vi "运维调试_CODCr.vi"() -> ()   [LabVIEW 2016, in "CodCr.lvlib"]
uses:
  CodCr.lvlib
  <vilib>/Utility/miscctls.llb/LVPointTypeDef.ctl
  <vilib>/Plasmionique/MB Master/MB_Master_Serial/MB_Master_Serial.lvclass
  C:/Program Files (x86)/National Instruments/LabVIEW 2016/vi.lib/Plasmionique/MB Master/MB_Master/MB_Master.lvclass
  <vilib>/Plasmionique/MB Master/MB Master.lvlib
  <vilib>/ptbypt/NI_PtbyPt.lvlib
panel:
  out "启动时间":timestamp format="%<%Y/%m/%d %H:%M:%S>T"
  out "?":errorcluster
  out "主循环次数":i32
  out "status":bool
  out "启动测量模式":T1(ring)
  out "曲线斜率B":sgl
  out "曲线斜率K":sgl
  out "量程上限":sgl
  out "量程下限":sgl
  out "消解时长":u16
  out "消解温度":u16
  out "测量精度":u16
  out "测量结果":sgl
  out "标样参考值":sgl
  out "量程":u16
  out "工作状态":T1(ring)
  out "仪器时间":timestamp format="%<%X\n%x>T"
  out "关键参数区":T2
  out "状态告警区":T3
  out "测量数据区":T4 {"单位" items=["ug/L", "mg/L", "ppm", "mg/m3", "cm", "ppb", "ug/m3", "%", "nmol/mol", "umol/mol", "MPN/L", "MPN/100ml", "ng/m3", "NTU", "无量纲", "ms/cm", "us/cm", "℃", "mV", "万个/L"]}
  out "error out":errorcluster
  out "系统时间":timestamp format="%<%Y/%m/%d %H:%M:%S>T"
  in  "VISA Resource":refnum<visa-resource-name>="COM9"
  out "Registers":u16[](array[numeric])
  in  "枚举":enum16{"读取", "写入", "读取参数"}(ring)
  in  "停止":bool
  in  "校时":bool
  in  "标样校准":bool
  in  "空白校准":bool
  in  "零点核查":bool
  in  "标样核查":bool
  in  "水样测试":bool
  in  "返回":bool
  in  "设置":bool
  # "mg/L"
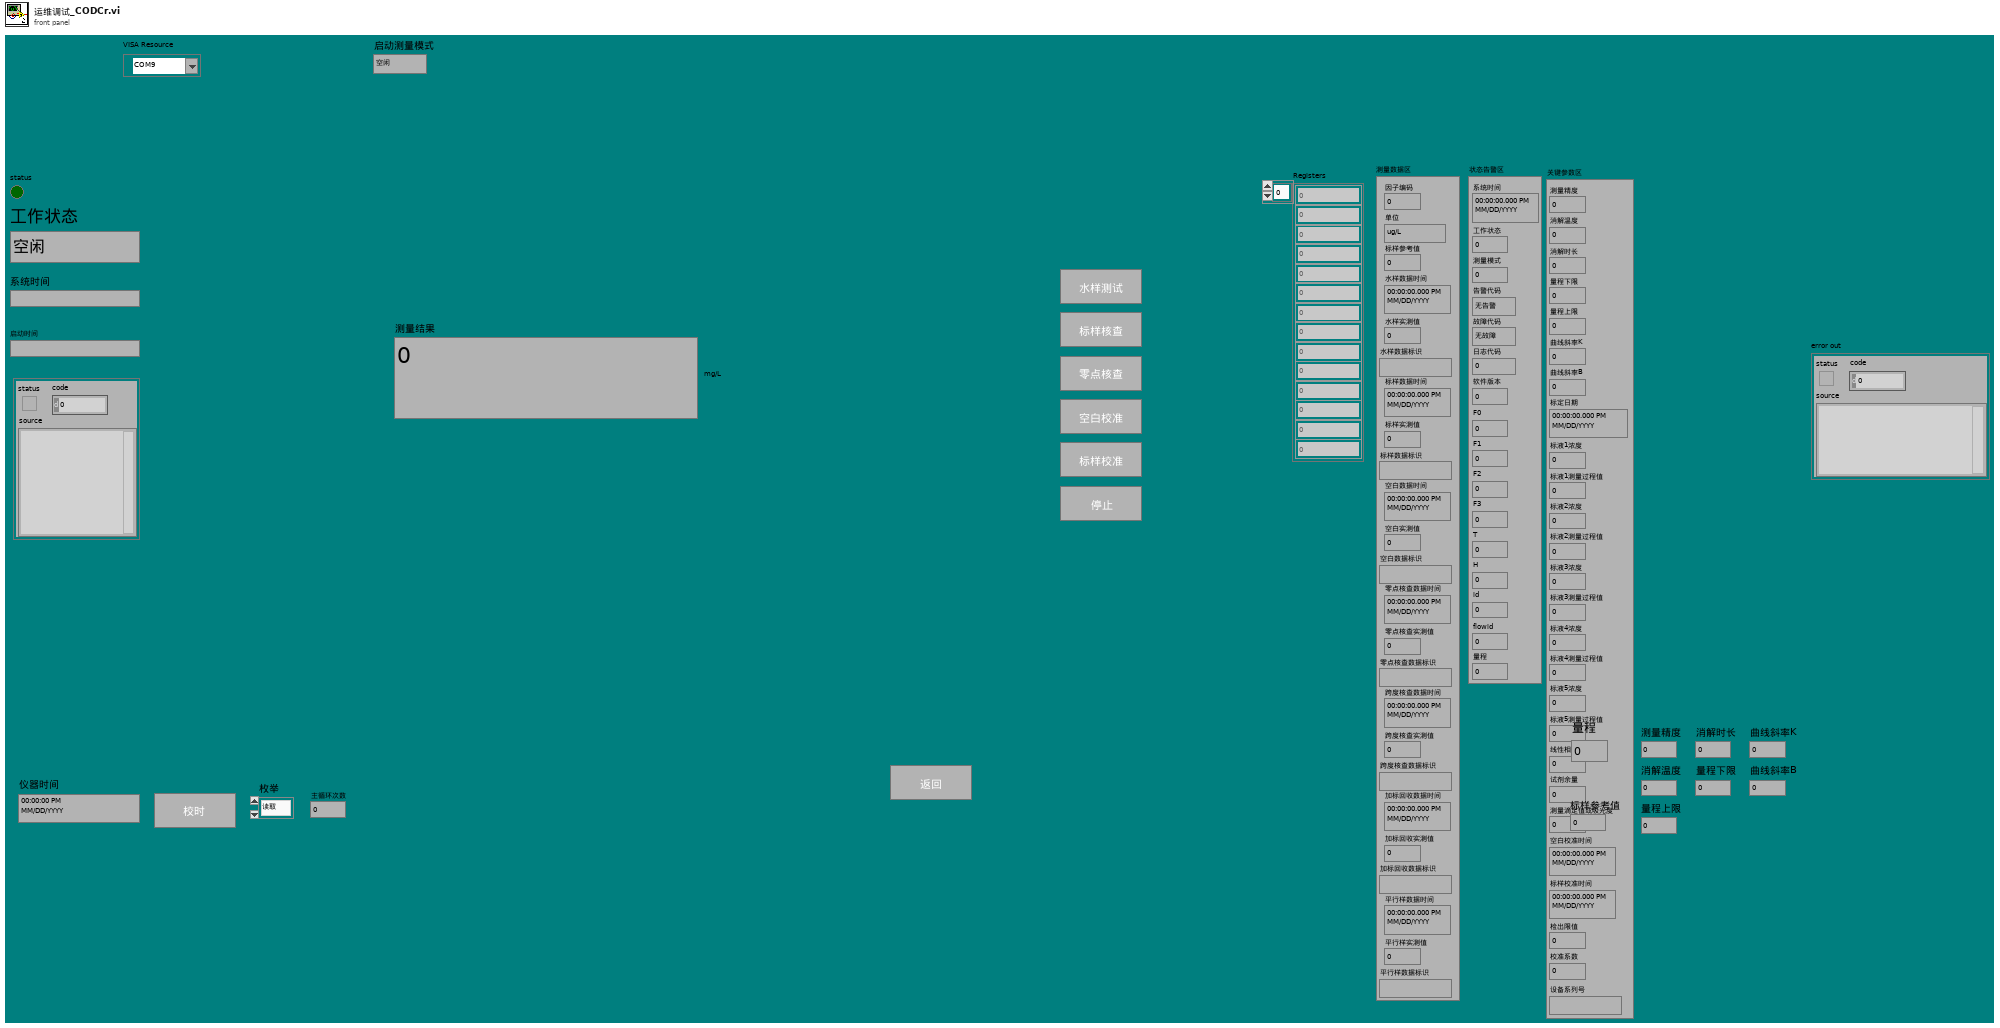
[diagram p1: front panel]
types:
  T1 = enum16{"空闲", "水样测试", "标样核查", "零点核查", "跨度核查", "空白测试", "平行样测试", "加标回收", "空白校准", "标样校准", "初始化（清洗）"}
  T2 = cluster{"测量精度":u16, "消解温度":u16, "消解时长":u16, "量程下限":sgl, "量程上限":sgl, "曲线斜率K":sgl, "曲线斜率B":sgl, "标定日期":timestamp, "标液1浓度":sgl, "标液1测量过程值":sgl, "标液2浓度":sgl, "标液2测量过程值":sgl, "标液3浓度":sgl, "标液3测量过程值":sgl, "标液4浓度":sgl, "标液4测量过程值":sgl, "标液5浓度":sgl, "标液5测量过程值":sgl, "线性相关系数":sgl, "试剂余量":u32, "测量滴定值或吸光度":sgl, "空白校准时间":timestamp, "标样校准时间":timestamp, "检出限值":sgl, "校准系数":sgl, "设备系列号":string}
  T3 = cluster{"系统时间":timestamp, "工作状态":u16, "测量模式":u16, "告警代码":enum16{"无告警", "缺试剂告警", "缺水样告警", "缺蒸馏水告警", "缺标液告警", "仪表漏液告警", "标定异常告警", "超量程告警", "加热异常", "低试剂预警", "超上限告警", "超下限告警", "仪表内部其他异常", "滴定异常告警", "电极异常告警", "量程切换告警", "参数设置告警", "PH电极电位异常", "电导率电极异常", "浊度光度异常", "溶解氧电极异常", "溶解氧光强异常", "温度异常告警", "PH异常告警", "溶解氧异常告警", "电导率异常告警", "浊度异常告警", "叶绿素异常告警", "藻密度异常告警", "蓝绿藻异常告警", "ORP异常告警", "氨氮异常告警", "清洁刷异常告警", "SD卡异常告警", "蓝牙异常告警", "Wifi异常告警", "流程异常告警"}, "故障代码":enum16{"无故障", "电机故障", "温度故障", "通讯故障", "滴定故障"}, "日志代码":u16, "软件版本":u16, "F0":sgl, "F1":sgl, "F2":sgl, "F3":sgl, "T":sgl, "H":sgl, "id":u16, "flowid":u16, "量程":u16}
  T4 = cluster{"因子编码":u32, "单位":u16, "标样参考值":sgl, "水样数据时间":timestamp, "水样实测值":sgl, "水样数据标识":string, "标样数据时间":timestamp, "标样实测值":sgl, "标样数据标识":string, "空白数据时间":timestamp, "空白实测值":sgl, "空白数据标识":string, "零点核查数据时间":timestamp, "零点核查实测值":sgl, "零点核查数据标识":string, "跨度核查数据时间":timestamp, "跨度核查实测值":sgl, "跨度核查数据标识":string, "加标回收数据时间":timestamp, "加标回收实测值":sgl, "加标回收数据标识":string, "平行样数据时间":timestamp, "平行样实测值":sgl, "平行样数据标识":string}
  T5 = cluster{"baud rate (bps)":u32, "stop bits":u16, "parity":u16, "flow control":u16, "timeout":u32, "retries":i32}
  T6 = cluster{"starting address":u16, "number of holding registers":u16}
  T7 = typedef "LVPointTypeDef.ctl" = cluster{"Horizontal":i16, "Vertical":i16}
  T8 = cluster{"时间标识":timestamp, "监测值":sgl, "单位":u16, "数据标识":string, "因子编码":u32, "标样参考值":sgl, "F0":sgl, "F1":sgl, "F2":sgl, "F3":sgl, "温度":sgl, "湿度":sgl, "量程标识":string}
  T9 = cluster{"系统时间":timestamp, "工作状态":enum16{"空闲", "水样测试", "标样核查", "零点核查", "跨度核查", "空白测试", "平行样测试", "加标回收", "空白校准", "标样校准", "初始化（清洗）"}, "测量模式":enum16{"待机", "连续模式", "周期模式", "定点模式", "受控模式", "手动模式"}, "告警代码":enum16{"无告警", "缺试剂告警", "缺水样告警", "缺蒸馏水告警", "缺标液告警", "仪表漏液告警", "标定异常告警", "超量程告警", "加热异常", "低试剂预警", "超上限告警", "超下限告警", "仪表内部其他异常", "滴定异常告警", "电极异常告警", "量程切换告警", "参数设置告警", "PH电极电位异常", "电导率电极异常", "浊度光度异常", "溶解氧电极异常", "溶解氧光强异常", "温度异常告警", "PH异常告警", "溶解氧异常告警", "电导率异常告警", "浊度异常告警", "叶绿素异常告警", "藻密度异常告警", "蓝绿藻异常告警", "ORP异常告警", "氨氮异常告警", "清洁刷异常告警", "SD卡异常告警", "蓝牙异常告警", "Wifi异常告警", "流程异常告警"}, "故障代码":enum16{"无故障", "电机故障", "温度故障", "通讯故障", "滴定故障"}, "日志代码":u16, "软件版本":u16, "F0":sgl, "F1":sgl, "F2":sgl, "F3":sgl, "T":sgl, "H":sgl, "id":u16, "flowid":u16, "量程":u16}
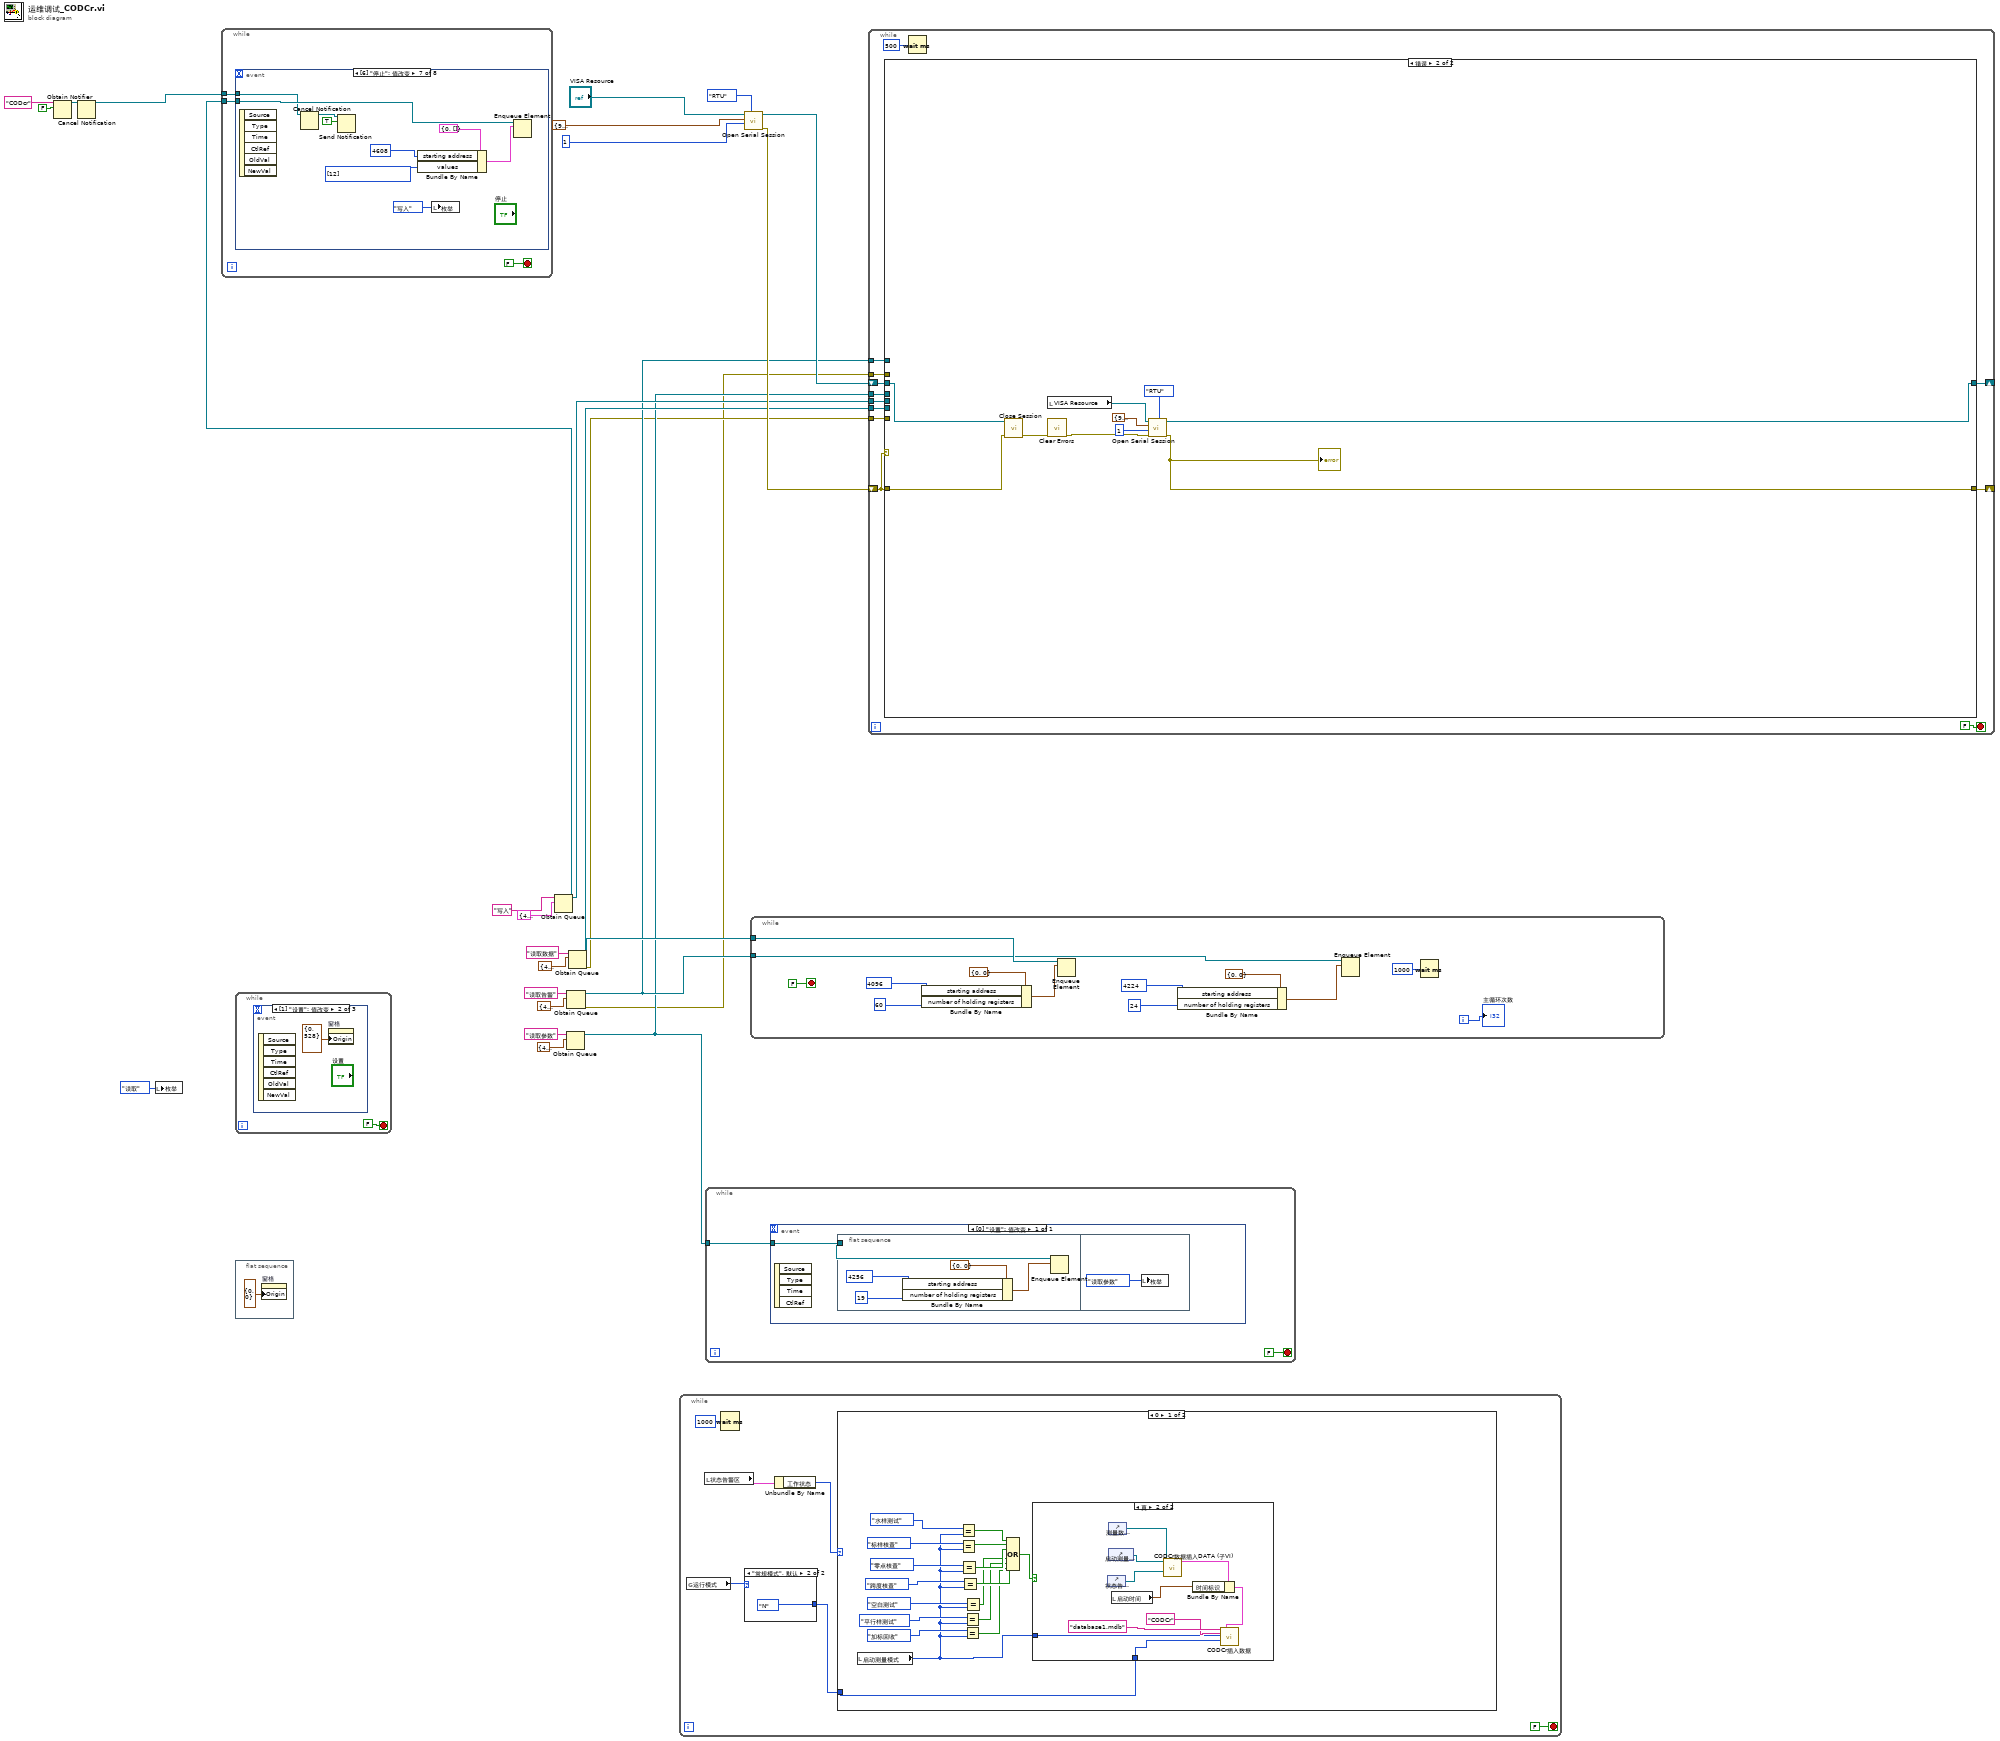
[diagram p0: block diagram]
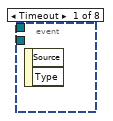
[diagram p2: hidden frame]
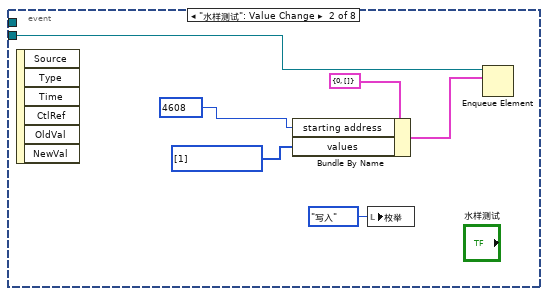
[diagram p3: hidden frame]
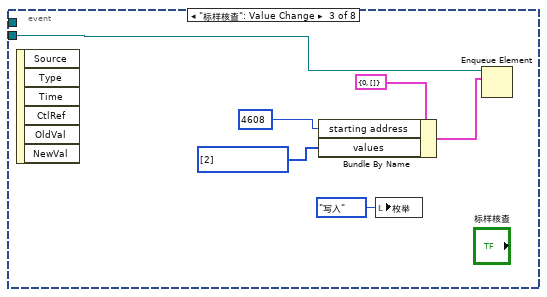
[diagram p4: hidden frame]
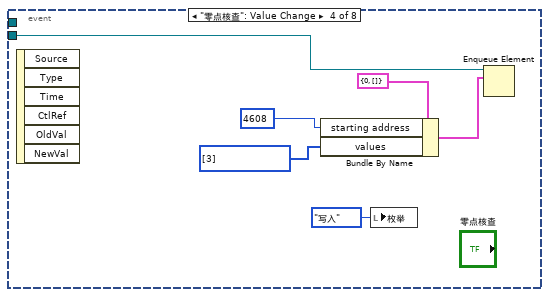
[diagram p5: hidden frame]
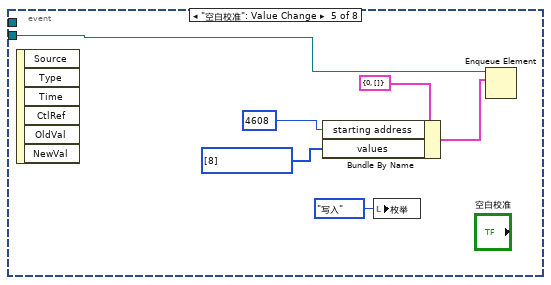
[diagram p6: hidden frame]
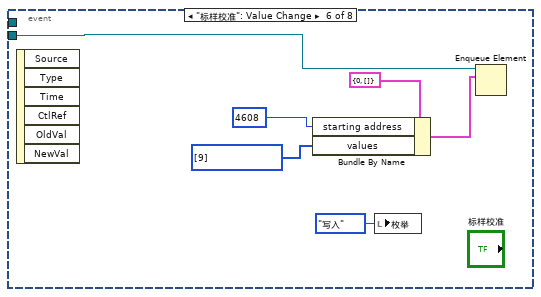
[diagram p7: hidden frame]
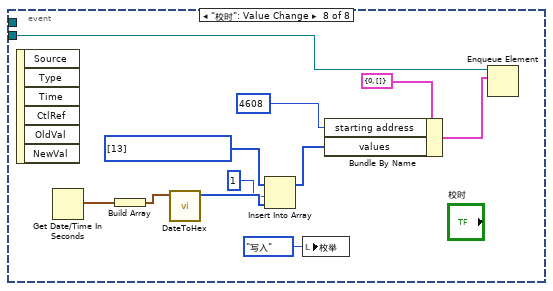
[diagram p8: hidden frame]
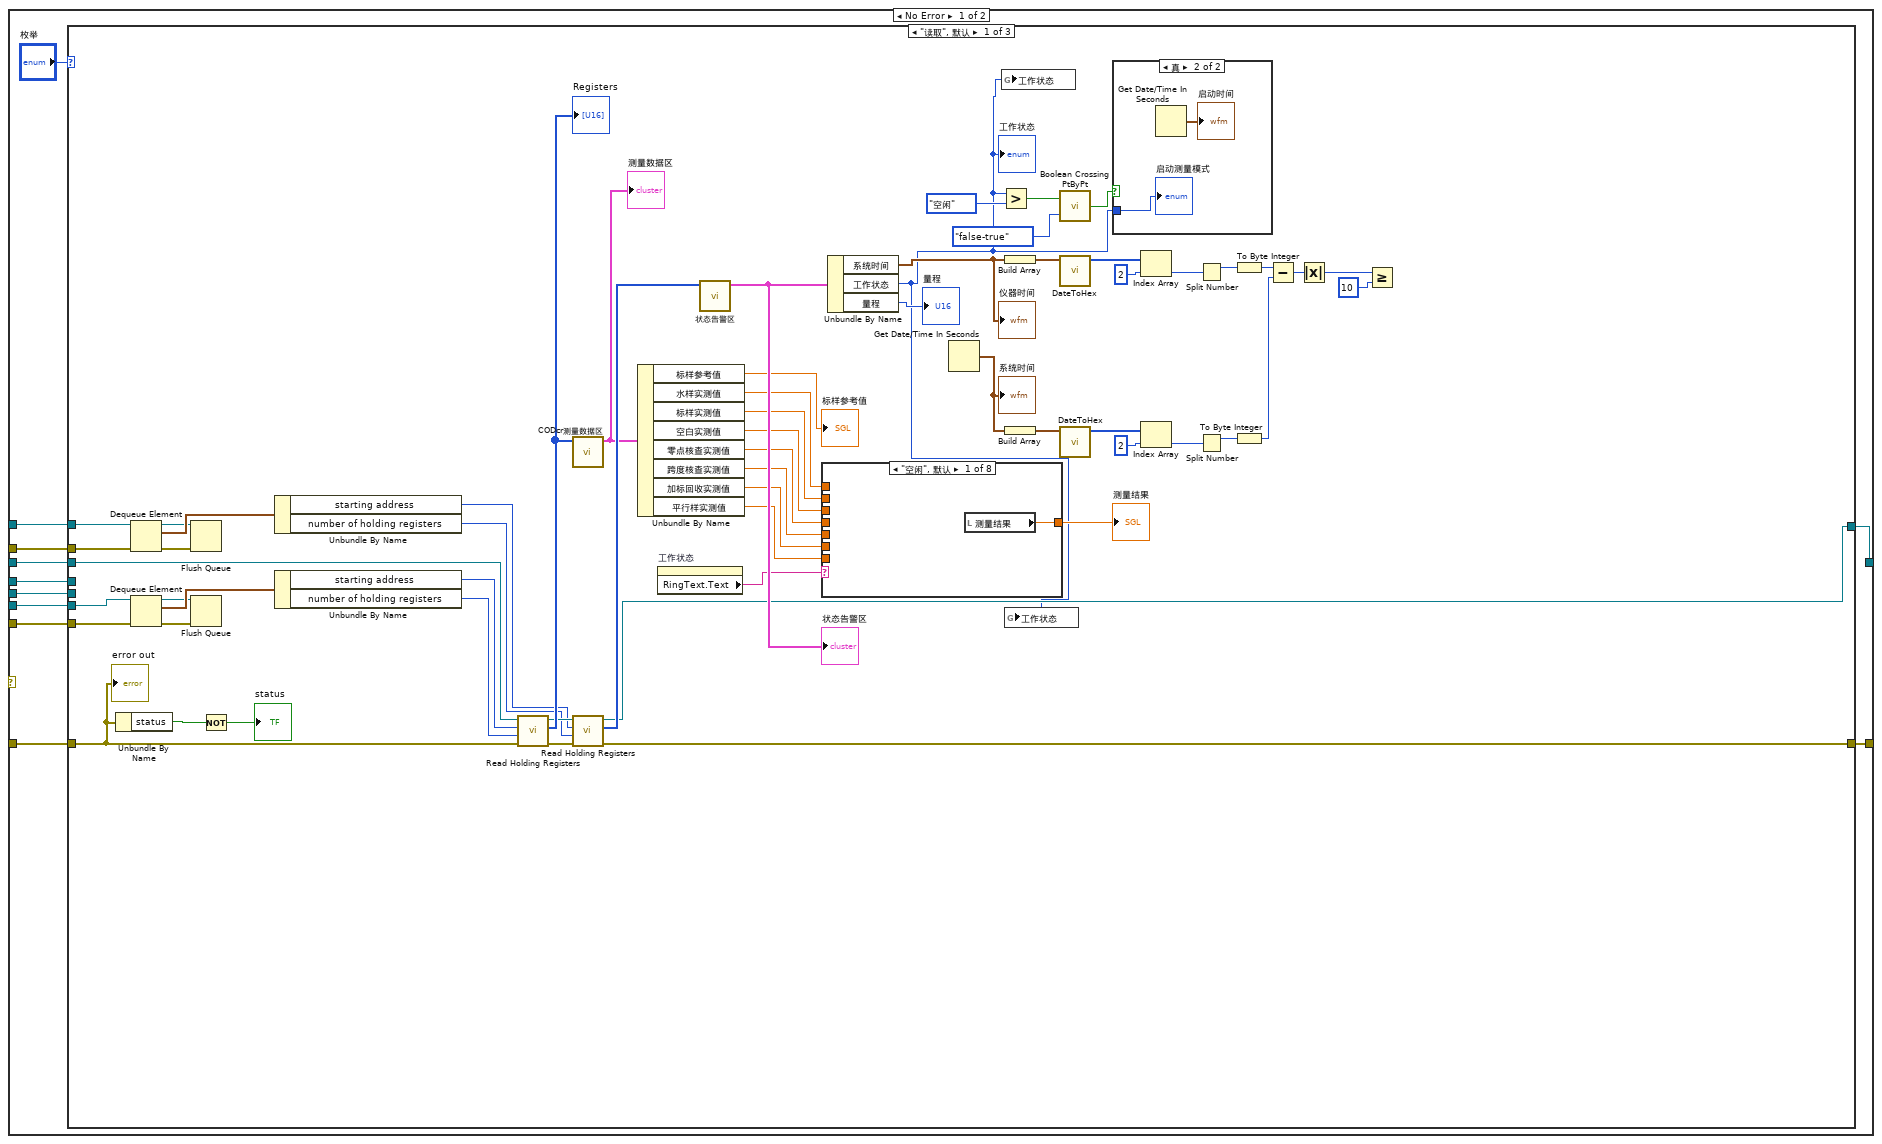
[diagram p9: hidden frame]
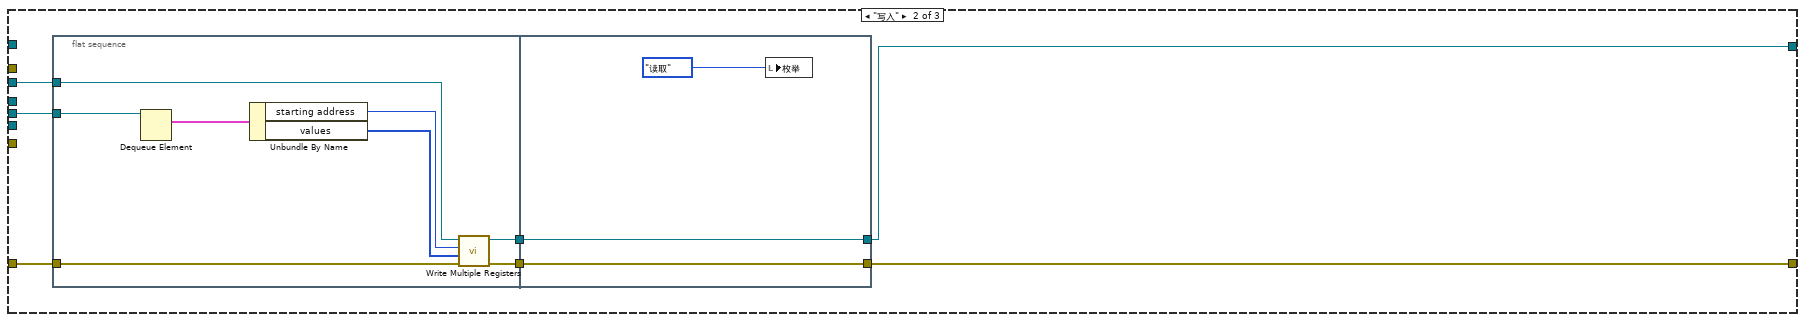
[diagram p18: hidden frame]
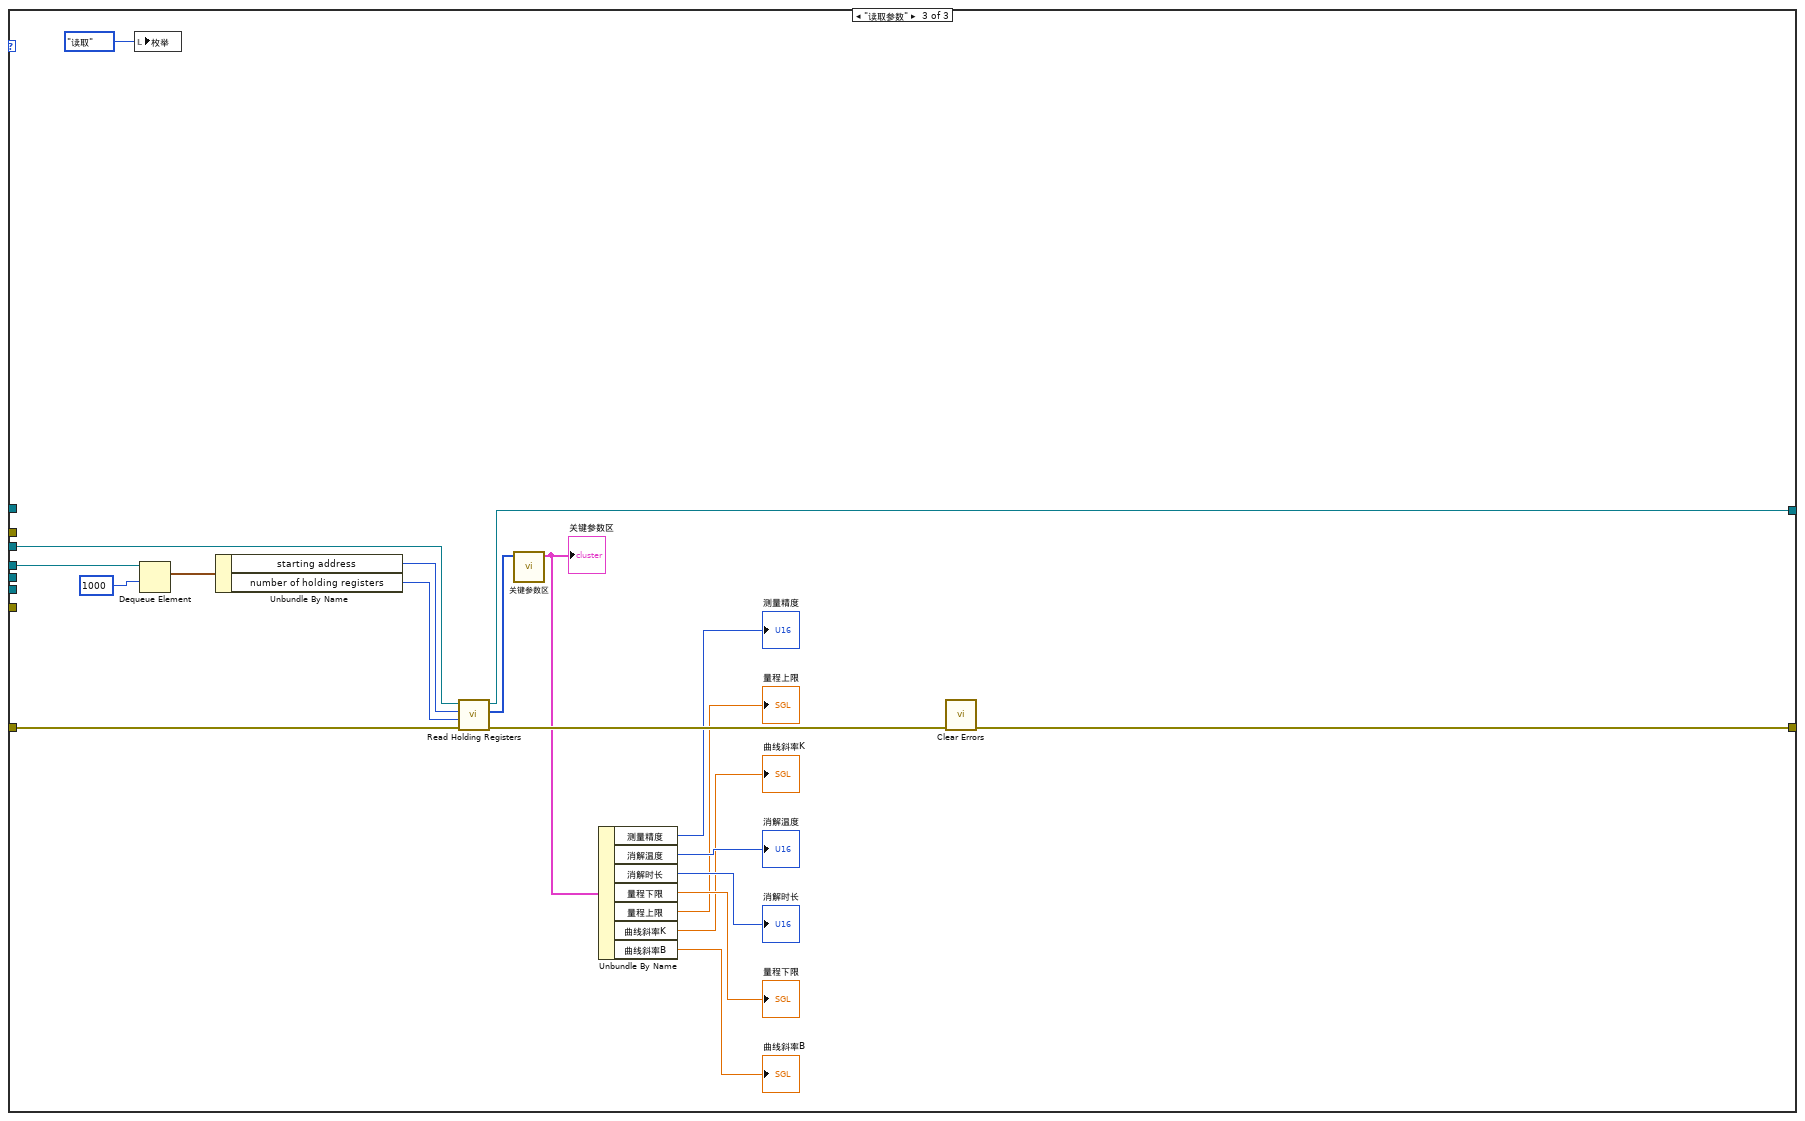
[diagram p19: hidden frame]
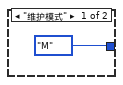
[diagram p20: hidden frame]
diagram:
  n1 = Obtain Notifier(name (unnamed)="CODcr" ("名称（未命名）"), notification data type=FALSE) -> (notifier out=w1:refnum<notifier>)  [unwired: 2 in, 2 out]
  n2 = Cancel Notification(0:w1) -> (8:w2:refnum<notifier>)  [unwired: 1 in, 2 out]
  n3 = local write "枚举"(enum16{"读取", "写入", "读取参数"}."读取" ("枚举")) -> ()
  n4 = while {
    stop <- FALSE stop-if-true
    n5 = event shown="[1] \"设置\": 值改变" {
      selector: _ -> [_ _ _]
      dyn-events: _ -> [_ _ _]
      timeout: _ -> [_ _ _]
      event Timeout {
        n6 = event-data() -> ()  [unwired: 1 in, 3 out]
      }
      event "设置": Value Change {
        n7 = event-data() -> ()  [unwired: 1 in, 6 out]
        n8 = property on="窗格" class="Pane"("Origin"=T7 {"Horizontal"=0, "Vertical"=528} ("原点")) -> ()  [unwired: 2 in, 2 out]
      }
      event "返回": Value Change {
        n9 = event-data() -> ()  [unwired: 1 in, 6 out]
        n10 = property on="窗格" class="Pane"("Origin"=T7 {"Horizontal"=0, "Vertical"=0} ("原点")) -> ()  [unwired: 2 in, 2 out]
      }
    }
  }
  n11 = flat-sequence {
    frame #0 {
      n12 = property on="窗格" class="Pane"("Origin"=T7 {"Horizontal"=0, "Vertical"=0} ("原点")) -> ()  [unwired: 2 in, 2 out]
    }
  }
  n13 = Obtain Queue(name (unnamed)="写入" ("名称（未命名）"), element data type=cluster{"starting address":u16, "values":u16[]} {"starting address"=4096, "values"=[]}) -> (queue out=w14:refnum<queue>)  [unwired: 3 in, 2 out]
  n14 = while {
    tunnel: w14 -> [w31]
    tunnel: w2 -> [w30]
    stop <- FALSE stop-if-true
    n15 = event shown="[6] \"停止\": 值改变" {
      selector: _ -> [_ _ _ _ _ _ _ _]
      dyn-events: _ -> [_ _ _ _ _ _ _ _]
      timeout: _ -> [_ _ _ _ _ _ _ _]
      tunnel: w31 -> [_ w38 w40 w46 w52 w58 w67 w79]
      tunnel: w30 -> [_ _ _ _ _ _ w65 _]
      event Timeout {
        n16 = event-data() -> ()  [unwired: 1 in, 2 out]
      }
      event "水样测试": Value Change {
        n17 = event-data() -> ()  [unwired: 1 in, 6 out]
        n18 = Bundle By Name(cluster=cluster{"starting address":u16, "values":u16[]} {"starting address"=0, "values"=[]} ("元素"), "starting address"=u16 4608, "values"=u16[] [1]) -> (w36:cluster{"starting address":u16, "values":u16[]})
        n19 = local write "枚举"(enum16{"读取", "写入", "读取参数"}."写入" ("枚举")) -> ()
        n20 = Enqueue Element(queue=w38, element=w36) -> ()  [unwired: 2 in, 3 out]
      }
      event "标样核查": Value Change {
        n21 = event-data() -> ()  [unwired: 1 in, 6 out]
        n22 = Bundle By Name(cluster=cluster{"starting address":u16, "values":u16[]} {"starting address"=0, "values"=[]} ("元素"), "starting address"=u16 4608, "values"=u16[] [2]) -> (w43:cluster{"starting address":u16, "values":u16[]})
        n23 = local write "枚举"(enum16{"读取", "写入", "读取参数"}."写入" ("枚举")) -> ()
        n24 = Enqueue Element(queue=w40, element=w43) -> ()  [unwired: 2 in, 3 out]
      }
      event "零点核查": Value Change {
        n25 = event-data() -> ()  [unwired: 1 in, 6 out]
        n26 = Bundle By Name(cluster=cluster{"starting address":u16, "values":u16[]} {"starting address"=0, "values"=[]} ("元素"), "starting address"=u16 4608, "values"=u16[] [3]) -> (w49:cluster{"starting address":u16, "values":u16[]})
        n27 = local write "枚举"(enum16{"读取", "写入", "读取参数"}."写入" ("枚举")) -> ()
        n28 = Enqueue Element(queue=w46, element=w49) -> ()  [unwired: 2 in, 3 out]
      }
      event "空白校准": Value Change {
        n29 = event-data() -> ()  [unwired: 1 in, 6 out]
        n30 = Bundle By Name(cluster=cluster{"starting address":u16, "values":u16[]} {"starting address"=0, "values"=[]} ("元素"), "starting address"=u16 4608, "values"=u16[] [8]) -> (w55:cluster{"starting address":u16, "values":u16[]})
        n31 = local write "枚举"(enum16{"读取", "写入", "读取参数"}."写入" ("枚举")) -> ()
        n32 = Enqueue Element(queue=w52, element=w55) -> ()  [unwired: 2 in, 3 out]
      }
      event "标样校准": Value Change {
        n33 = event-data() -> ()  [unwired: 1 in, 6 out]
        n34 = Bundle By Name(cluster=cluster{"starting address":u16, "values":u16[]} {"starting address"=0, "values"=[]} ("元素"), "starting address"=u16 4608, "values"=u16[] [9]) -> (w61:cluster{"starting address":u16, "values":u16[]})
        n35 = local write "枚举"(enum16{"读取", "写入", "读取参数"}."写入" ("枚举")) -> ()
        n36 = Enqueue Element(queue=w58, element=w61) -> ()  [unwired: 2 in, 3 out]
      }
      event "停止": Value Change {
        n37 = event-data() -> ()  [unwired: 1 in, 6 out]
        n38 = Cancel Notification(0:w65) -> (8:w64:refnum<notifier>)  [unwired: 1 in, 2 out]
        n39 = Send Notification(notification=TRUE ("通知"), notifier=w64) -> ()  [unwired: 1 in, 2 out]
        n40 = Bundle By Name(cluster=cluster{"starting address":u16, "values":u16[]} {"starting address"=0, "values"=[]} ("元素"), "starting address"=u16 4608, "values"=u16[] [12]) -> (w70:cluster{"starting address":u16, "values":u16[]})
        n41 = local write "枚举"(enum16{"读取", "写入", "读取参数"}."写入" ("枚举")) -> ()
        n42 = Enqueue Element(queue=w67, element=w70) -> ()  [unwired: 2 in, 3 out]
      }
      event "校时": Value Change {
        n43 = event-data() -> ()  [unwired: 1 in, 6 out]
        n44 = Get Date/Time In Seconds() -> (seconds since 1Jan1904=w78:timestamp)
        n45 = Build Array(w78) -> (w77:timestamp[])
        n46 = call "DateToHex.vi"("DATE"=w77) -> ("数组"=w75:u16[])  [unwired: 10 in]
        n47 = Insert Into Array(array=u16[] [13] ("values"), index=1 ("索引"), new element=w75) -> (w73:u16[])
        n48 = local write "枚举"(enum16{"读取", "写入", "读取参数"}."写入" ("枚举")) -> ()
        n49 = Bundle By Name(cluster=cluster{"starting address":u16, "values":u16[]} {"starting address"=0, "values"=[]} ("元素"), "starting address"=u16 4608, "values"=w73) -> (w81:cluster{"starting address":u16, "values":u16[]})
        n50 = Enqueue Element(queue=w79, element=w81) -> ()  [unwired: 2 in, 3 out]
      }
    }
  }
  n51 = Obtain Queue(name (unnamed)="读取参数" ("名称（未命名）"), element data type=T6 {"starting address"=4096, "number of holding registers"=100}) -> (queue out=w8:refnum<queue>)  [unwired: 3 in, 2 out]
  n52 = Obtain Queue(name (unnamed)="读取告警" ("名称（未命名）"), element data type=T6 {"starting address"=4096, "number of holding registers"=100}) -> (queue out=w11:refnum<queue>, error out=w5:errorcluster)  [unwired: 3 in, 1 out]
  n53 = Obtain Queue(name (unnamed)="读取数据" ("名称（未命名）"), element data type=T6 {"starting address"=4096, "number of holding registers"=100}) -> (queue out=w15:refnum<queue>, error out=w6:errorcluster)  [unwired: 3 in, 1 out]
  n54 = while {
    stop <- FALSE stop-if-true
    n55 = global read "系统变量.vi" "运行模式"() -> (w84:enum16{"维护模式", "常规模式", "应急模式", "质控模式"})
    n56 = local read "状态告警区"() -> (w86:T3)
    n57 = Wait (ms)(milliseconds to wait=u32 1000 ("等待时间（毫秒）")) -> ()  [unwired: 1 out]
    n58 = case shown="\"常规模式\", 默认" w84 {
      tunnel: [enum16{"N", "M"}."M" ("数据类型") enum16{"N", "M"}."N" ("数据类型")] -> w83
      frame "维护模式" {
      }
      frame "常规模式", Default {
      }
    }
    n59 = Unbundle By Name(w86) -> ("工作状态"=w85:u16)
    n60 = case shown="0" w85 {
      tunnel: w83 -> [w107 _]
      frame 0 {
        n61 = local read "启动测量模式"() -> (w99:T1)
        n62 = Equal?(x=T1."水样测试" ("启动测量模式"), y=w99) -> (x = y?=w98:bool)
        n63 = Equal?(x=T1."标样核查" ("启动测量模式"), y=w99) -> (x = y?=w97:bool)
        n64 = Equal?(x=T1."零点核查" ("启动测量模式"), y=w99) -> (x = y?=w96:bool)
        n65 = Equal?(x=T1."跨度核查" ("启动测量模式"), y=w99) -> (x = y?=w95:bool)
        n66 = Equal?(x=T1."平行样测试" ("启动测量模式"), y=w99) -> (x = y?=w93:bool)
        n67 = Equal?(x=T1."加标回收" ("启动测量模式"), y=w99) -> (x = y?=w92:bool)
        n68 = Equal?(x=T1."空白测试" ("启动测量模式"), y=w99) -> (x = y?=w94:bool)
        n69 = Compound Arithmetic op=OR(w98, w97, w96, w95, w94, w93, w92) -> (w91:bool)
        n70 = case shown="真" w91 {
          tunnel: w99 -> [_ w115]
          tunnel: w107 -> [_ w114]
          frame False {
          }
          frame True {
            n71 = control-ref of="状态告警区"() -> (w111:refnum<vi>)
            n72 = control-ref of="启动测量模式"() -> (w113:refnum<vi>)
            n73 = control-ref of="测量数据区"() -> (w112:refnum<vi>)
            n74 = local read "启动时间"() -> (w109:timestamp)
            n75 = call "CODCr数据插入DATA (子VI).vi"("reference 2"=w111, "reference"=w112, "Enum输入"=w113) -> ("data"=w110:T8)  [unwired: 8 in]
            n76 = Bundle By Name(cluster=w110, "时间标识"=w109) -> (w108:T8)
            n77 = call "CODCr插入数据.vi"("database"="database1.mdb", "data"=w108, "table"="CODCr", "测量模式"=w115, "数据类型"=w114) -> ()  [unwired: 10 in, 1 out]
          }
        }
      }
      frame 1, Default {
      }
    }
  }
  n78 = while {
    tunnel: w8 -> [w118]
    stop <- FALSE stop-if-true
    n79 = event shown="[0] \"设置\": 值改变" {
      selector: _ -> [_]
      dyn-events: _ -> [_]
      timeout: _ -> [_]
      tunnel: w118 -> [w120]
      event "设置": Value Change {
        n80 = event-data() -> ()  [unwired: 1 in, 4 out]
        n81 = flat-sequence {
          tunnel: w120 -> [w121]
          frame #0 {
            n82 = Bundle By Name(cluster=T6 {"starting address"=0, "number of holding registers"=0} ("元素"), "starting address"=u16 4256, "number of holding registers"=u16 19) -> (w125:T6)
            n83 = Enqueue Element(queue=w121, element=w125) -> ()  [unwired: 2 in, 3 out]
          }
          frame #1 {
            n84 = local write "枚举"(enum16{"读取", "写入", "读取参数"}."读取参数" ("枚举")) -> ()
          }
        }
      }
    }
  }
  n85 = call <vilib>:"Open Serial Session.vi"("Mode (RTU)"=enum16{"RTU", "ASCII"}."RTU", "Slave ID"=u8 1, "Serial Config"=T5 {"baud rate (bps)"=9600, "stop bits"=10, "parity"=0, "flow control"=0, "timeout"=1000, "retries"=1}, "VISA Resource"="VISA Resource") -> ("Error out"=w24:errorcluster, "MB_Serial session"=w25:refnum<class "MB_Master_Serial.lvclass">)  [unwired: 6 in]
  n86 = while {
    tunnel: w15 -> [w137]
    tunnel: w11 -> [w128]
    i -> [w127]
    stop <- FALSE stop-if-true
    n87 = Bundle By Name(cluster=T6 {"starting address"=0, "number of holding registers"=0} ("元素"), "starting address"=u16 4096, "number of holding registers"=u16 60) -> (w135:T6)
    n88 = Enqueue Element(queue=w137, element=w135) -> ()  [unwired: 2 in, 3 out]
    n89 = Bundle By Name(cluster=T6 {"starting address"=0, "number of holding registers"=0} ("元素"), "starting address"=u16 4224, "number of holding registers"=u16 24) -> (w129:T6)
    n90 = Enqueue Element(queue=w128, element=w129) -> ()  [unwired: 2 in, 3 out]
    n91 = Wait (ms)(milliseconds to wait=u32 1000 ("等待时间（毫秒）")) -> ()  [unwired: 1 out]
    "主循环次数" <- w127
  }
  n92 = while {
    tunnel: w14 -> [w148]
    tunnel: w15 -> [w147]
    tunnel: w11 -> [w146]
    tunnel: w8 -> [w145]
    shift-right: [w143] -> _
    shift-left: w25 -> [w149]
    shift-right: [w144] -> _
    shift-left: w24 -> [w140]
    tunnel: w6 -> [w142]
    tunnel: w5 -> [w141]
    stop <- FALSE stop-if-true
    n93 = case shown="错误" w140 {
      tunnel: w149 -> [w162 w277]
      tunnel: w140 -> [w161 w276]
      tunnel: w148 -> [w160 _]
      tunnel: w147 -> [w159 _]
      tunnel: w146 -> [w158 _]
      tunnel: w145 -> [w156 _]
      tunnel: [w155 w270] -> w144
      tunnel: [w154 w271] -> w143
      tunnel: w142 -> [w153 _]
      tunnel: w141 -> [w152 _]
      frame No Error {
        n94 = case shown="\"读取\", 默认" "枚举" {
          tunnel: w162 -> [w221 w238 w261]
          tunnel: w161 -> [w194 w237 w260]
          tunnel: w160 -> [_ w236 _]
          tunnel: w159 -> [w220 _ _]
          tunnel: w158 -> [w215 _ _]
          tunnel: w156 -> [_ _ w262]
          tunnel: [w191 w232 w250] -> w155
          tunnel: [w173 w233 w251] -> w154
          tunnel: w153 -> [w167 _ _]
          tunnel: w152 -> [w164 _ _]
          frame "读取", Default {
            n95 = Unbundle By Name(w194) -> ("status"=w193:bool)
            n96 = Dequeue Element(queue=w215, error in (no error)=w164) -> (queue out=w166:refnum<queue>, element=w214:T6, error out=w165:errorcluster)  [unwired: 1 in, 1 out]
            n97 = Dequeue Element(queue=w220, error in (no error)=w167) -> (queue out=w169:refnum<queue>, element=w219:T6, error out=w168:errorcluster)  [unwired: 1 in, 1 out]
            n98 = Flush Queue(queue=w166, error in (no error)=w165) -> ()  [unwired: 3 out]
            n99 = Flush Queue(queue=w169, error in (no error)=w168) -> ()  [unwired: 3 out]
            n100 = Not(x=w193) -> (.not. x?=→"status":bool)
            n101 = Unbundle By Name(w214) -> ("starting address"=w211:u16, "number of holding registers"=w210:u16)
            n102 = Unbundle By Name(w219) -> ("starting address"=w218:u16, "number of holding registers"=w217:u16)
            n103 = call <vilib>:"Read Holding Registers.vi"("error in (no error)"=w194, "quantity"=w217, "starting address"=w218, "MB session in"=w221) -> ("error out"=w212:errorcluster, "Registers"=w216:u16[], "MB session out"=w213:refnum<class "MB_Master_Serial.lvclass">)  [unwired: 5 in]
            "Registers" <- w216
            n104 = call "CODcr测量数据区.vi"("数组"=w216) -> ("测量数据区"=w206:T4)  [unwired: 10 in]
            "测量数据区" <- w206
            n105 = call <vilib>:"Read Holding Registers.vi"("error in (no error)"=w212, "quantity"=w210, "starting address"=w211, "MB session in"=w213) -> ("error out"=w191:errorcluster, "Registers"=w209:u16[], "MB session out"=w173:refnum<class "MB_Master_Serial.lvclass">)  [unwired: 5 in]
            n106 = Unbundle By Name(w206) -> ("标样参考值"=→"标样参考值":sgl, "水样实测值"=w202:sgl, "标样实测值"=w200:sgl, "空白实测值"=w197:sgl, "零点核查实测值"=w199:sgl, "跨度核查实测值"=w198:sgl, "加标回收实测值"=w195:sgl, "平行样实测值"=w196:sgl)
            n107 = property on="工作状态" class="Enum (严格)"() -> ("RingText.Text"=w203:string)  [unwired: 2 in, 2 out]
            n108 = call "状态告警区.vi"("数组"=w209) -> ("状态告警区"=w208:T9)  [unwired: 10 in]
            "状态告警区" <- w208
            n109 = case shown="\"空闲\", 默认" w203 {
              tunnel: w202 -> [_ w223 _ _ _ _ _ _]
              tunnel: [w222 w223 w224 w225 w226 w227 w228 w229] -> w201
              tunnel: w200 -> [_ _ w224 _ _ _ _ _]
              tunnel: w199 -> [_ _ _ w225 _ _ _ _]
              tunnel: w198 -> [_ _ _ _ w226 _ _ _]
              tunnel: w197 -> [_ _ _ _ _ w227 _ _]
              tunnel: w196 -> [_ _ _ _ _ _ w228 _]
              tunnel: w195 -> [_ _ _ _ _ _ _ w229]
              frame "空闲", Default {
                n110 = local read "测量结果"() -> (w222:sgl)
              }
              frame "水样测试" {
              }
              frame "标样核查" {
              }
              frame "零点核查" {
              }
              frame "跨度核查" {
              }
              frame "空白测试" {
              }
              frame "平行样测试" {
              }
              frame "加标回收" {
              }
            }
            "测量结果" <- w201
            n111 = Unbundle By Name(w208) -> ("系统时间"=w174:timestamp, "工作状态"=w163:T1, "量程"=→"量程":u16)
            "仪器时间" <- w174
            "工作状态" <- w163
            n112 = Get Date/Time In Seconds() -> (seconds since 1Jan1904=w176:timestamp)
            "系统时间" <- w176
            n113 = Greater?(x=w163, y=T1."空闲") -> (0:w172:bool)
            n114 = global write "CODcr全局变量.vi" "工作状态"(w163) -> ()
            n115 = Build Array(w174) -> (w190:timestamp[])
            n116 = Build Array(w176) -> (w175:timestamp[])
            n117 = global write "CODCr工作状态.vi" "工作状态"(w163) -> ()
            n118 = call <vilib>:"Boolean Crossing PtByPt.vi"("direction"=enum16{"either", "false-true", "true-false"}."false-true", "input"=w172) -> ("crossing"=w171:bool)  [unwired: 1 in]
            n119 = call "DateToHex.vi"("DATE"=w190) -> ("数组"=w182:u16[])  [unwired: 10 in]
            n120 = call "DateToHex.vi"("DATE"=w175) -> ("数组"=w177:u16[])  [unwired: 10 in]
            n121 = case shown="真" w171 {
              tunnel: w163 -> [_ w231]
              frame False {
              }
              frame True {
                n122 = Get Date/Time In Seconds() -> (seconds since 1Jan1904=→"启动时间":timestamp)
                "启动测量模式" <- w231
              }
            }
            n123 = Index Array(array=w182, index=2 ("索引")) -> (element=w180:u16)
            n124 = Index Array(array=w177, index=2 ("索引")) -> (element=w179:u16)
            n125 = Split Number(x=w180) -> (hi(x)=w186:u8)  [unwired: 1 out]
            n126 = Split Number(x=w179) -> (hi(x)=w183:u8)  [unwired: 1 out]
            n127 = To Byte Integer(number=w186) -> (8bit integer=w187:i8)
            n128 = To Byte Integer(number=w183) -> (8bit integer=w184:i8)
            n129 = Subtract(x=w187, y=w184) -> (x-y=w185:i8)
            n130 = Absolute Value(x=w185) -> (abs(x)=w188:i8)
            n131 = Greater Or Equal?(x=w188, y=i8 10) -> ()  [unwired: 1 out]
            "error out" <- w194
          }
          frame "写入" {
            n132 = flat-sequence {
              tunnel: w238 -> [w246]
              tunnel: w237 -> [w245]
              tunnel: w236 -> [w242]
              tunnel: [w244] -> w235
              tunnel: [w243] -> w234
              tunnel: w235 -> [w248]
              tunnel: w234 -> [w247]
              tunnel: [w248] -> w233
              tunnel: [w247] -> w232
              frame #0 {
                n133 = Dequeue Element(queue=w242) -> (element=w241:cluster{"starting address":u16, "values":u16[]})  [unwired: 2 in, 3 out]
                n134 = Unbundle By Name(w241) -> ("starting address"=w240:u16, "values"=w239:u16[])
                n135 = call <vilib>:"Write Multiple Registers.vi"("error in (no error)"=w245, "values"=w239, "starting address"=w240, "MB session in"=w246) -> ("error out"=w243:errorcluster, "MB session out"=w244:refnum<class "MB_Master_Serial.lvclass">)  [unwired: 6 in]
              }
              frame #1 {
                n136 = local write "枚举"(enum16{"读取", "写入", "读取参数"}."读取" ("枚举")) -> ()
              }
            }
          }
          frame "读取参数" {
            n137 = local write "枚举"(enum16{"读取", "写入", "读取参数"}."读取" ("枚举")) -> ()
            n138 = Dequeue Element(queue=w262, timeout in ms (-1)=1000 ("超时毫秒(-1)")) -> (element=w269:T6)  [unwired: 1 in, 3 out]
            n139 = Unbundle By Name(w269) -> ("starting address"=w268:u16, "number of holding registers"=w267:u16)
            n140 = call <vilib>:"Read Holding Registers.vi"("error in (no error)"=w260, "quantity"=w267, "starting address"=w268, "MB session in"=w261) -> ("error out"=w264:errorcluster, "Registers"=w266:u16[], "MB session out"=w251:refnum<class "MB_Master_Serial.lvclass">)  [unwired: 5 in]
            n141 = call "关键参数区.vi"("数组"=w266) -> ("关键参数区"=w263:T2)  [unwired: 10 in]
            "关键参数区" <- w263
            n142 = Unbundle By Name(w263) -> ("测量精度"=→"测量精度":u16, "消解温度"=→"消解温度":u16, "消解时长"=→"消解时长":u16, "量程下限"=→"量程下限":sgl, "量程上限"=→"量程上限":sgl, "曲线斜率K"=→"曲线斜率K":sgl, "曲线斜率B"=→"曲线斜率B":sgl)
            n143 = call <vilib>:"Clear Errors.vi"("error in (no error)"=w264) -> ("error out"=w250:errorcluster)  [unwired: 5 in, 1 out]
          }
        }
      }
      frame Error {
        n144 = call-dynamic "Close Session.vi"("error in (no error)"=w276, "MB_Serial session"=w277) -> ("error out"=w275:errorcluster)  [unwired: 9 in]
        n145 = local read "VISA Resource"() -> (w273:refnum<visa-resource-name>)
        n146 = call <vilib>:"Clear Errors.vi"("error in (no error)"=w275) -> ("error out"=w274:errorcluster)  [unwired: 5 in, 1 out]
        n147 = call <vilib>:"Open Serial Session.vi"("Mode (RTU)"=enum16{"RTU", "ASCII"}."RTU", "Error in"=w274, "Slave ID"=u8 1, "Serial Config"=T5 {"baud rate (bps)"=9600, "stop bits"=10, "parity"=0, "flow control"=0, "timeout"=1000, "retries"=1}, "VISA Resource"=w273) -> ("Error out"=w270:errorcluster, "MB_Serial session"=w271:refnum<class "MB_Master_Serial.lvclass">)  [unwired: 5 in]
        "?" <- w270
      }
    }
    n148 = Wait (ms)(milliseconds to wait=u32 500 ("等待时间（毫秒）")) -> ()  [unwired: 1 out]
  }
